vi "ColumbiaSonicareStby.vi"() -> ()   [LabVIEW 2022 SP3]
uses:
  Doppler data processing/Doppler/dopplerV6.llb/AI Waveform Scan (waveform).vi
  Doppler data processing/Doppler/dopplerV6.llb/AI Read (waveform).vi
  <vilib>/sound/lvsound.llb/Sound Format.ctl
panel:
  in  "Mode":enum32{"HIFU", "Thromb"}(tab)
  out "Exp Count":i32
  in  "Time between exposures (s)":sgl=2.2 min=0 format="%.1f"
  in  "Number of Exposures":i32=1 min=1
  in  "Therapy Duration (s)":dbl=0.1 min=0.1 max=10.0 step=0.1 format="%.1f"
  out "Time":i32=1 min=1
  out "PRF time  (ms)":sgl format="%.3f"
  in  "exp per cycle  (ms)":sgl=0.5 format="%.3f"
  in  "Total  Time On (s)":sgl=1.0 min=0.001 format="%.2f"
  out "PRF  (kHz)":sgl=1.0 min=0.001 format="%.3f"
  in  "Duty Cycle":sgl=0.5 min=0 max=1 format="%.2f"
  in  "EKG ?":bool=TRUE
  in  "Re-Zero Trig":bool
  out "waveform data":waveform(dbl)[](array[waveform])
  in  "New EKG (F1)":bool
  in  "Exit Program (F2)":bool
  out "EKG":waveform(dbl)[](graph)
  in  "Fire Therapy (ESC)":bool
  out "Therapy Delay (s)":dbl=1.0 format="%.3f"
  # "1. Select EKG mode with switch below.\n2. If in EKG mode, update EKG trace with New EKG (F1).\n3. Drag pink line to mark start time of exposure and trigger level.\n4. Set time duration of exposure (0.1 s steps).\n5. Choose number of exposures and time between exposures (2.2 s min in EKG mode)..\n6. Start exposure with Fire Therapy (ESC) (Green means on).\n7. Press Fire Therapy (ESC) again for emergency stop (Red means off).\n8. To exit program, Press Exit Program (F2) to  terminate program.\n9. Thromb tab permits exposures of a fixed PRF, duty cycle, and time duration. EKG  is\n     inactive when Thromb is selected."
  # "© 2003 Riverside Research Institute"
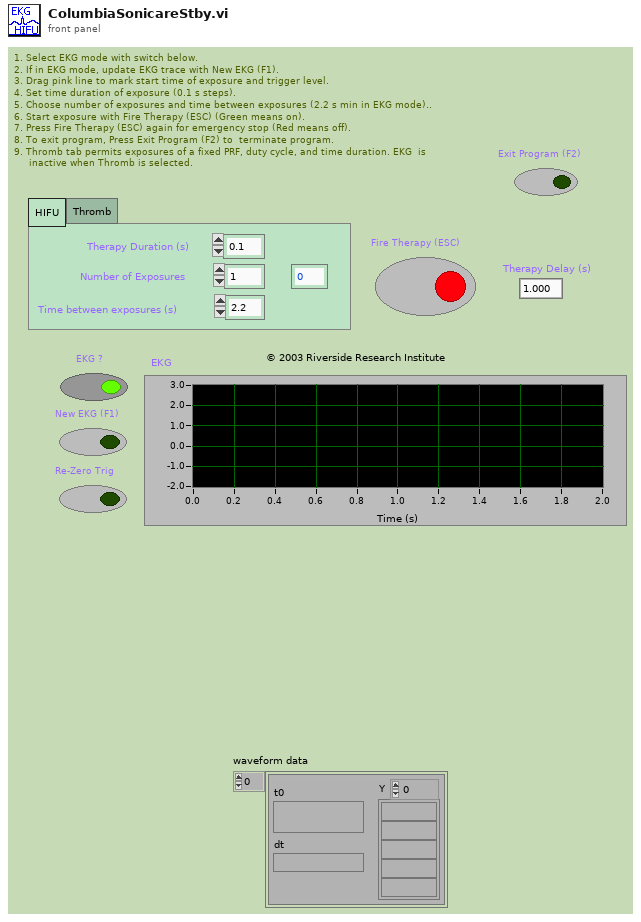
[diagram p1: front panel]
types:
  T1 = cluster{"coupling (no change:0)":enum16{"no change", "DC", "AC", "GND", "internal ref."}, "input config (no change:0)":u16}[]
  T2 = cluster{"high limit (0.0)":sgl, "low limit (0.0)":sgl}[]
  T3 = cluster{"trigger type (no trig:0)":enum16{"no trigger", "analog", "digital A", "digital B", "scan clock gate", "software analog "}, "pretrigger scans (0)":i32, "edge or slope \n(no change)":enum16{"no change", "rising", "falling"}, "analog chan (-) & level (0.0)":cluster{"trigger channel (empty)":string, "level (0.0)":sgl}, "scan clock source\n(no change:0)":enum16{"no change", "internal", "I/O Connector", "RTSI"}}
  T4 = typedef "Sound Format.ctl" = cluster{"sound quality":enum16{"mono", "stereo"}, "rate":enum16{"11025", "22050", "44100", "8000"}, "bits per sample":enum16{"8 bit", "16 bit"}}
  T5 = enum16{"ungated/software start", "count while high", "count while low", "start on rising edge", "start on falling edge"}
  T6 = enum16{"no trigger", "analog", "digital A", "digital A & B", "scan clock gate"}
  T7 = cluster{"trigger channel (empty)":string, "Cursor.Cursor Y":dbl}
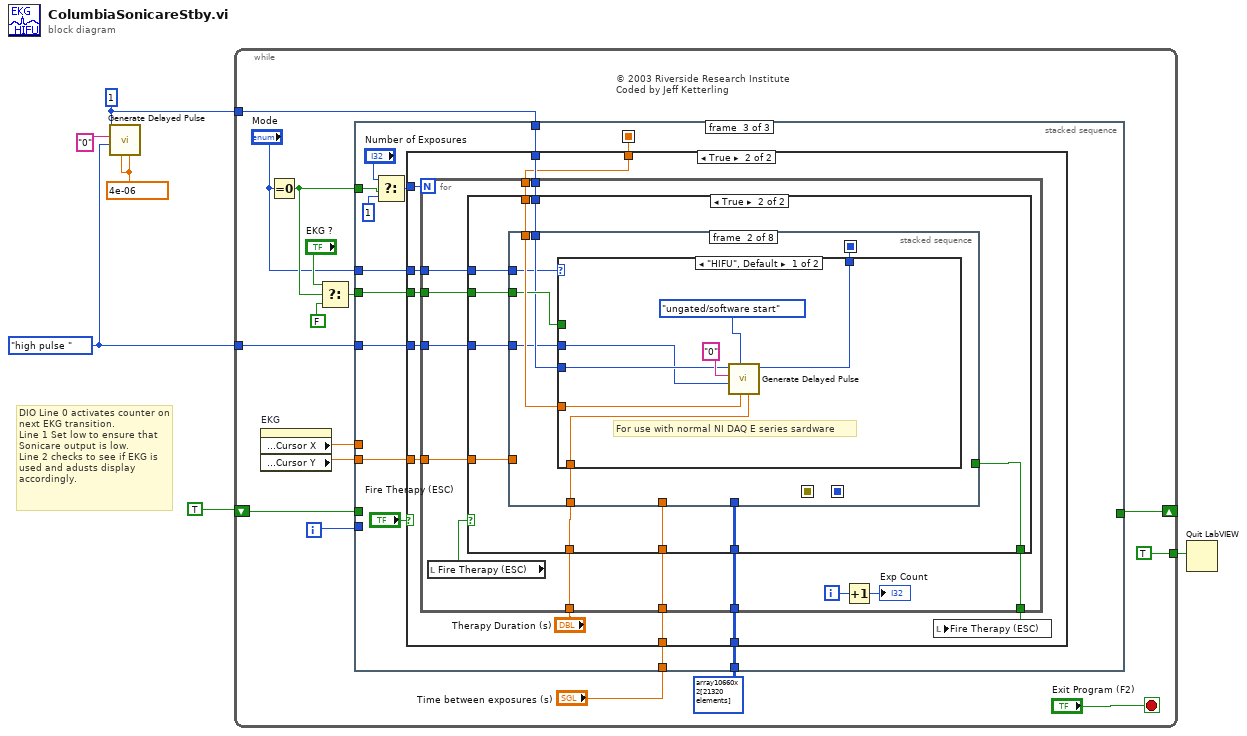
[diagram p0: block diagram]
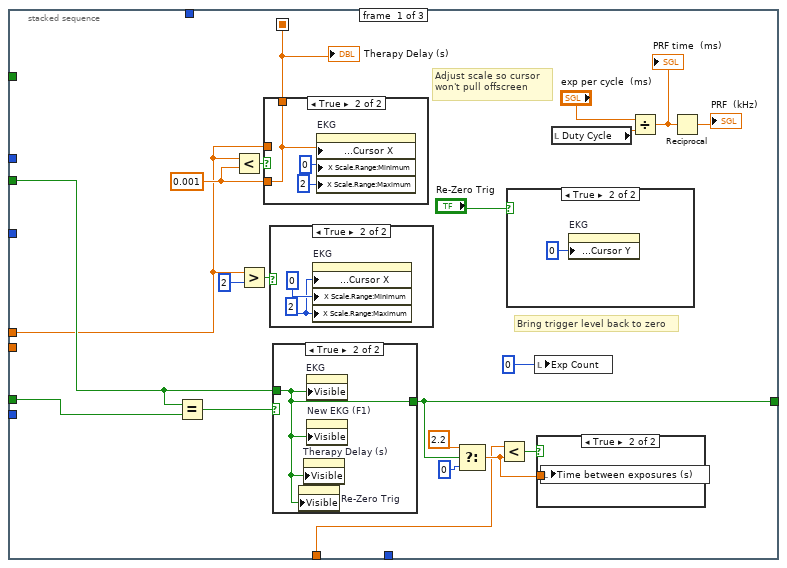
[diagram p2: hidden frame]
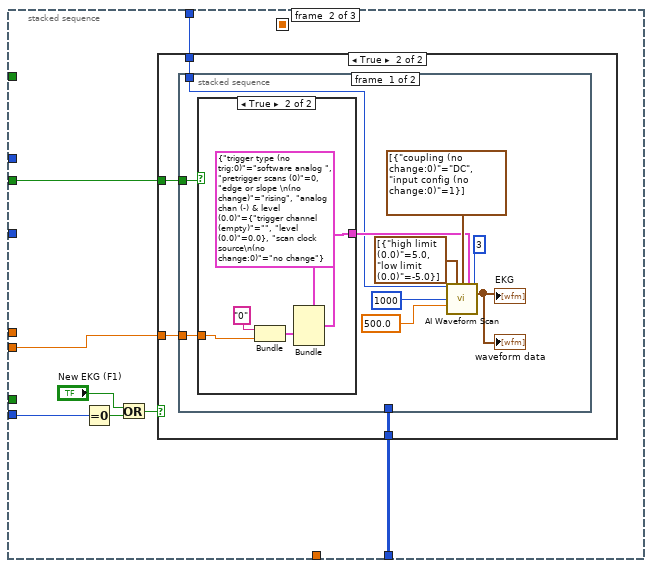
[diagram p8: hidden frame]
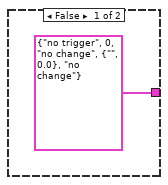
[diagram p10: hidden frame]
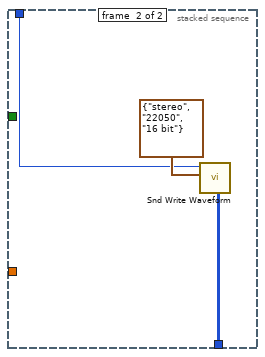
[diagram p11: hidden frame]
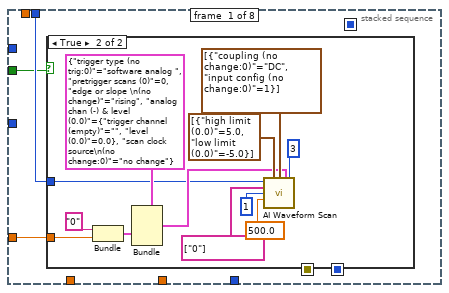
[diagram p14: hidden frame]
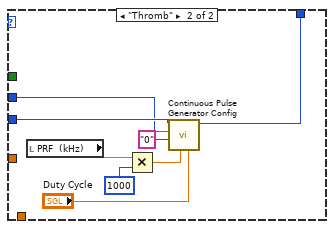
[diagram p16: hidden frame]
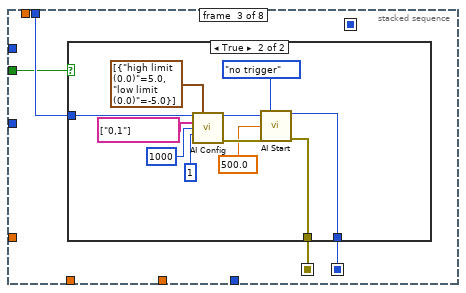
[diagram p17: hidden frame]
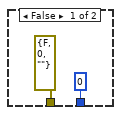
[diagram p18: hidden frame]
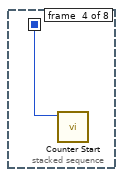
[diagram p19: hidden frame]
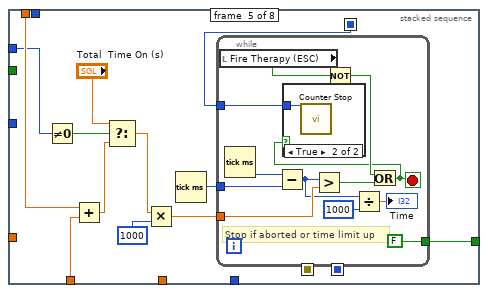
[diagram p20: hidden frame]
diagram:
  w2 = enum16{"high pulse ", "low pulse"}."high pulse " ("pulse polarity (high:0)")
  w3 = 4e-06
  w1 = 1
  # "DIO Line 0 activates counter on next EKG transition.\nLine 1 Set low to ensure that Sonicare output is low.\nLine 2 checks to see if EKG is used and adusts display accordingly."
  n1 = call <vilib>:"Generate Delayed Pulse.vi"("pulse width (s or cycles)"=w3, "pulse delay (s or cycles)"=w3, "pulse polarity (high:0)"=w2, "counter"="0", "device"=w1) -> ()  [unwired: 4 in, 3 out]
  n2 = while {
    tunnel: w1 -> [w18]
    shift-right: [w19] -> _
    shift-left: TRUE -> [w20]
    tunnel: [TRUE] -> w5
    tunnel: w2 -> [w7]
    i -> [w21]
    stop <- "Exit Program (F2)" stop-if-true
    # "© 2003 Riverside Research Institute\nCoded by Jeff Ketterling"
    n3 = property on="EKG" class="WFGraph (strict)"() -> ("Cursor.Cursor Position:Cursor X"=w15:dbl, "Cursor.Cursor Position:Cursor Y"=w16:dbl)  [unwired: 2 in, 2 out]
    n4 = Equal To 0?(x="Mode") -> (x = 0?=w9:bool)
    n5 = Select(t="EKG ?", s=w9, f=FALSE) -> (s? t:f=w11:bool)
    n6 = stacked-sequence {
      seq-local: [w42 _ _] -> [_ _ w95]
      tunnel: w18 -> [_ w61 w97]
      tunnel: w21 -> [_ w60 _]
      tunnel: w11 -> [w38 w56 w96]
      tunnel: w20 -> [w37 _ _]
      tunnel: [w29 _ _] -> w19
      tunnel: w16 -> [_ w55 w94]
      tunnel: w15 -> [w35 _ _]
      tunnel: i16[][] array10660x2[21320 elements] ("stereo 16-bit") -> [_ w54 w93]
      tunnel: "Time between exposures (s)" -> [w28 _ w92]
      tunnel: w9 -> [_ _ w89]
      tunnel: "Mode" -> [_ _ w86]
      tunnel: w7 -> [_ _ w85]
      frame #0 {
        w41 = 0.001
        # "Bring trigger level back to zero"
        # "Adjust scale so cursor won't pull offscreen"
        n7 = Equal?(x=w38, y=w37) -> (x = y?=w36:bool)
        n8 = Less?(x=w35, y=w41) -> (x < y?=w43:bool)
        n9 = Greater?(x=w35, y=2) -> (0:w39:bool)
        n10 = case shown="True" w43 {
          tunnel: w35 -> [w50 _]
          tunnel: [w50 w53] -> w42
          tunnel: w41 -> [_ w53]
          frame False {
          }
          frame True {
            n11 = property on="EKG" class="WFGraph (strict)"("Cursor.Cursor Position:Cursor X"=w53, "X Scale.Range:Minimum"=0, "X Scale.Range:Maximum"=2) -> ()  [unwired: 2 in, 2 out]
          }
        }
        "Therapy Delay (s)" <- w42
        n12 = case shown="True" w39 {
          frame False {
          }
          frame True {
            w48 = 2
            n13 = property on="EKG" class="WFGraph (strict)"("Cursor.Cursor Position:Cursor X"=w48, "X Scale.Range:Minimum"=0, "X Scale.Range:Maximum"=w48) -> ()  [unwired: 2 in, 2 out]
          }
        }
        n14 = case shown="True" w36 {
          tunnel: w38 -> [w46 w47]
          tunnel: [w46 w47] -> w29
          frame False {
          }
          frame True {
            n15 = property on="Re-Zero Trig" class="Bool"("Visible"=w47) -> ()  [unwired: 2 in, 2 out]
            n16 = property on="Therapy Delay (s)" class="DigNum (strict)"("Visible"=w47) -> ()  [unwired: 2 in, 2 out]
            n17 = property on="EKG" class="WFGraph (strict)"("Visible"=w47) -> ()  [unwired: 2 in, 2 out]
            n18 = property on="New EKG (F1)" class="Bool"("Visible"=w47) -> ()  [unwired: 2 in, 2 out]
          }
        }
        n19 = Select(t=2.2, s=w29, f=0) -> (s? t:f=w30:dbl)
        n20 = Less?(x=w28, y=w30) -> (x < y?=w31:bool)
        n21 = case shown="True" "Re-Zero Trig" {
          frame False {
          }
          frame True {
            n22 = property on="EKG" class="WFGraph (strict)"("Cursor.Cursor Position:Cursor Y"=0) -> ()  [unwired: 2 in, 2 out]
          }
        }
        n23 = local write "Exp Count"(0) -> ()
        n24 = case shown="True" w31 {
          tunnel: w30 -> [_ w44]
          frame False {
          }
          frame True {
            n25 = local write "Time between exposures (s)"(w44) -> ()
          }
        }
        n26 = local read "Duty Cycle"() -> (w26:sgl)
        n27 = Divide(x="exp per cycle  (ms)", y=w26) -> (x/y=w24:sgl)
        "PRF time  (ms)" <- w24
        n28 = Reciprocal(x=w24) -> (1/x=→"PRF  (kHz)":sgl)
      }
      frame #1 {
        n29 = Equal To 0?(x=w60) -> (x = 0?=w59:bool)
        n30 = Or(x="New EKG (F1)", y=w59) -> (x .or. y?=w57:bool)
        n31 = case shown="True" w57 {
          tunnel: w61 -> [_ w64]
          tunnel: w56 -> [_ w65]
          tunnel: w55 -> [_ w63]
          tunnel: w54 -> [_ w62]
          frame False {
          }
          frame True {
            n32 = stacked-sequence {
              tunnel: w65 -> [w68 _]
              tunnel: w64 -> [w67 w82]
              tunnel: w63 -> [w66 _]
              tunnel: w62 -> [_ w83]
              frame #0 {
                n33 = case shown="True" w68 {
                  tunnel: [T3 {"trigger type (no trig:0)"=enum."no trigger", "pretrigger scans (0)"=0, "edge or slope \n(no change)"=enum."no change", "analog chan (-) & level (0.0)"={"trigger channel (empty)"="", "level (0.0)"=0.0}, "scan clock source\n(no change:0)"=enum."no change"} ("trigger and clock (no trig, int clk)") w81] -> w70
                  tunnel: w66 -> [_ w80]
                  frame False {
                  }
                  frame True {
                    n34 = Bundle("trigger channel (empty)"="0", "Cursor.Cursor Y"=w80) -> (w78:T7)  [unwired: 1 in]
                    n35 = Bundle(cluster=T3 {"trigger type (no trig:0)"=enum."software analog ", "pretrigger scans (0)"=0, "edge or slope \n(no change)"=enum."rising", "analog chan (-) & level (0.0)"={"trigger channel (empty)"="", "level (0.0)"=0.0}, "scan clock source\n(no change:0)"=enum."no change"} ("trigger and clock (no trig, int clk)"), "analog chan (-) & level (0.0)"=w78) -> (w81:T3)  [unwired: 4 in]
                  }
                }
                n36 = call-poly "AI Waveform Scan.vi"("device (1)"=w67, "input limits (no change)"=T2 [{"high limit (0.0)"=5.0, "low limit (0.0)"=-5.0}], "coupling & input config (no change:0)"=T1 [{"coupling (no change:0)"=enum."DC", "input config (no change:0)"=1}], "trigger and clock (no trig, int clk)"=w70, "time limit in sec \n(computed:-1)"=3, "number of scans\n(1000)"=1000, "scan rate (1000 scans/sec)"=sgl 500.0) -> ("waveform data"=→"EKG" →"waveform data":waveform(dbl)[])  [unwired: 7 in, 1 out]
              }
              frame #1 {
                n37 = call <vilib>:"Snd Write Waveform.vi"("stereo 16-bit"=w83, "sound format"=T4 {"sound quality"=enum."stereo", "rate"=enum."22050", "bits per sample"=enum."16 bit"}, "device (0)"=w82) -> ()  [unwired: 8 in, 1 out]
              }
            }
          }
        }
      }
      frame #2 {
        n38 = Select(t="Number of Exposures", s=w89, f=1) -> (s? t:f=w87:i32)
        n39 = case shown="True" "Fire Therapy (ESC)" {
          tunnel: w97 -> [_ w108]
          tunnel: w96 -> [_ w107]
          tunnel: w95 -> [_ w106]
          tunnel: w87 -> [_ w105]
          tunnel: w94 -> [_ w104]
          tunnel: w93 -> [_ w102]
          tunnel: w92 -> [_ w101]
          tunnel: w86 -> [_ w99]
          tunnel: w85 -> [_ w98]
          frame False {
          }
          frame True {
            n40 = for {
              N: w105 -> [_]
              tunnel: w108 -> [w121]
              tunnel: w106 -> [w120]
              tunnel: w107 -> [w119]
              tunnel: w104 -> [w118]
              tunnel: [w117] -> w103
              tunnel: w102 -> [w116]
              tunnel: w101 -> [w114]
              tunnel: "Therapy Duration (s)" -> [w113]
              tunnel: w99 -> [w110]
              tunnel: w98 -> [w109]
              i -> [w115]
              n41 = local read "Fire Therapy (ESC)"() -> (w111:bool)
              n42 = case shown="True" w111 {
                selector: w111 -> [w122 _]
                tunnel: w121 -> [_ w132]
                tunnel: w120 -> [_ w131]
                tunnel: w119 -> [_ w130]
                tunnel: w118 -> [_ w129]
                tunnel: [w122 w128] -> w117
                tunnel: w116 -> [_ w127]
                tunnel: w114 -> [_ w126]
                tunnel: w113 -> [_ w125]
                tunnel: w110 -> [_ w124]
                tunnel: w109 -> [_ w123]
                frame False {
                }
                frame True {
                  n43 = stacked-sequence {
                    seq-local: [_ w151 _ _ _ _ _ _] -> [_ _ _ w187 w193 _ _ _]
                    seq-local: [_ _ w172 _ _ _ _ _] -> [_ _ _ _ _ w215 _ _]
                    seq-local: [_ _ w171 _ _ _ _ _] -> [_ _ _ _ _ w214 _ _]
                    tunnel: w132 -> [w135 w150 w173 _ _ _ w222 _]
                    tunnel: [_ _ _ _ w196 _ _ _] -> w128
                    tunnel: w131 -> [_ w154 _ _ w195 _ _ _]
                    tunnel: w125 -> [_ w153 _ _ w194 _ _ _]
                    tunnel: w130 -> [w134 w152 w170 _ _ w213 _ w227]
                    tunnel: w129 -> [w133 _ _ _ _ _ _ _]
                    tunnel: w127 -> [_ _ _ _ _ _ w223 _]
                    tunnel: w126 -> [_ _ _ _ _ _ _ w225]
                    tunnel: w124 -> [_ w149 _ _ w190 _ _ _]
                    tunnel: w123 -> [_ w148 _ _ _ _ _ _]
                    frame #0 {
                      n44 = case shown="True" w134 {
                        tunnel: w135 -> [_ w137]
                        tunnel: w133 -> [_ w138]
                        frame False {
                        }
                        frame True {
                          n45 = Bundle("trigger channel (empty)"="0", "Cursor.Cursor Y"=w138) -> (w139:T7)  [unwired: 1 in]
                          n46 = Bundle(cluster=T3 {"trigger type (no trig:0)"=enum."software analog ", "pretrigger scans (0)"=0, "edge or slope \n(no change)"=enum."rising", "analog chan (-) & level (0.0)"={"trigger channel (empty)"="", "level (0.0)"=0.0}, "scan clock source\n(no change:0)"=enum."no change"} ("trigger and clock (no trig, int clk)"), "analog chan (-) & level (0.0)"=w139) -> (w141:T3)  [unwired: 4 in]
                          n47 = call-poly "AI Waveform Scan.vi"("device (1)"=w137, "input limits (no change)"=T2 [{"high limit (0.0)"=5.0, "low limit (0.0)"=-5.0}], "coupling & input config (no change:0)"=T1 [{"coupling (no change:0)"=enum."DC", "input config (no change:0)"=1}], "trigger and clock (no trig, int clk)"=w141, "time limit in sec \n(computed:-1)"=3, "channels (0)"=tag[] ["0"], "number of scans\n(1000)"=1, "scan rate (1000 scans/sec)"=sgl 500.0) -> ()  [unwired: 6 in, 2 out]
                        }
                      }
                    }
                    frame #1 {
                      n48 = case shown="\"HIFU\", Default" w149 {
                        tunnel: w154 -> [w160 _]
                        tunnel: w153 -> [w159 _]
                        tunnel: w152 -> [_ _]
                        tunnel: [w158 w167] -> w151
                        tunnel: w150 -> [w157 w168]
                        tunnel: w148 -> [w155 w162]
                        frame "HIFU", Default {
                          # "For use with normal NI DAQ E series sardware"
                          n49 = call <vilib>:"Generate Delayed Pulse.vi"("pulse width (s or cycles)"=w159, "pulse delay (s or cycles)"=w160, "gate mode (ungated:0)"=T5."ungated/software start", "pulse polarity (high:0)"=w155, "counter"="0", "device"=w157) -> ("[taskID]"=w158:u32)  [unwired: 3 in, 2 out]
                        }
                        frame "Thromb" {
                          n50 = local read "PRF  (kHz)"() -> (w163:sgl)
                          n51 = Multiply(x=w163, y=1000) -> (x*y=w165:sgl)
                          n52 = call <vilib>:"Continuous Pulse Generator Config.vi"("duty cycle (0.5)"="Duty Cycle", "frequency (Hz)"=w165, "pulse polarity (high:0)"=w162, "counter"="0", "device"=w168) -> ("taskID"=w167:u32)  [unwired: 3 in, 3 out]
                        }
                      }
                    }
                    frame #2 {
                      n53 = case shown="True" w170 {
                        tunnel: w173 -> [_ w179]
                        tunnel: [u32 0 ("taskID out") w178] -> w172
                        tunnel: [errorcluster {"status"=FALSE, "code"=0, "source"=""} ("error out") w177] -> w171
                        frame False {
                        }
                        frame True {
                          n54 = call "AI Config.vi"("device (1)"=w179, "input limits (no change)"=T2 [{"high limit (0.0)"=5.0, "low limit (0.0)"=-5.0}], "channels (0)"=tag[] ["0,1"], "buffer size (1000 scans)"=1000, "[group] (0)"=1) -> ("taskID"=w181:u32, "error out"=w186:errorcluster)  [unwired: 8 in, 1 out]
                          n55 = call "AI Start.vi"("taskID in"=w181, "trigger type (no trig:0)"=T6."no trigger", "scan rate (1000 scans/sec)"=sgl 500.0, "error in (no error)"=w186) -> ("taskID out"=w178:u32, "error out"=w177:errorcluster)  [unwired: 8 in, 2 out]
                        }
                      }
                    }
                    frame #3 {
                      n56 = call <vilib>:"Counter Start.vi"("taskID"=w187) -> ()  [unwired: 9 in, 2 out]
                    }
                    frame #4 {
                      n57 = Not Equal To 0?(x=w190) -> (x != 0?=w192:bool)
                      n58 = Add(x=w195, y=w194) -> (x+y=w189:dbl)
                      n59 = Select(t="Total  Time On (s)", s=w192, f=w189) -> (s? t:f=w188:dbl)
                      n60 = Multiply(x=w188, y=1000) -> (x*y=w197:dbl)
                      n61 = Tick Count (ms)() -> (millisecond timer value=w199:u32)
                      n62 = while {
                        tunnel: w193 -> [w211]
                        tunnel: w199 -> [w209]
                        tunnel: w197 -> [w208]
                        tunnel: [FALSE] -> w196
                        stop <- w203 stop-if-true
                        # "Stop if aborted or time limit up"
                        n63 = local read "Fire Therapy (ESC)"() -> (w205:bool)
                        n64 = Tick Count (ms)() -> (millisecond timer value=w210:u32)
                        n65 = Subtract(x=w210, y=w209) -> (x-y=w202:u32)
                        n66 = Greater?(x=w202, y=w208) -> (0:w207:bool)
                        n67 = Not(x=w205) -> (.not. x?=w204:bool)
                        n68 = Divide(x=w202, y=1000) -> (x/y=→"Time":dbl)
                        n69 = Or(x=w204, y=w207) -> (x .or. y?=w203:bool)
                        n70 = case shown="True" w203 {
                          tunnel: w211 -> [_ w212]
                          frame False {
                          }
                          frame True {
                            n71 = call <vilib>:"Counter Stop.vi"("taskID"=w212) -> ()  [unwired: 5 in, 2 out]
                          }
                        }
                      }
                    }
                    frame #5 {
                      n72 = case shown="True" w213 {
                        tunnel: w215 -> [_ w217]
                        tunnel: w214 -> [_ w216]
                        frame False {
                        }
                        frame True {
                          n73 = call-poly "AI Read.vi"("taskID in"=w217, "number of scans to read (-1:all)"=1000, "error in (no error)"=w216) -> ("taskID out"=w220:u32, "waveform data"=w218:waveform(dbl)[], "error out"=w219:errorcluster)  [unwired: 7 in, 3 out]
                          n74 = local write "EKG"(w218) -> ()
                          n75 = call "AI Clear.vi"("error in (no error)"=w219, "taskID in"=w220) -> ()  [unwired: 4 in, 2 out]
                        }
                      }
                    }
                    frame #6 {
                      n76 = call <vilib>:"Snd Write Waveform.vi"("stereo 16-bit"=w223, "sound format"=T4 {"sound quality"=enum."stereo", "rate"=enum."22050", "bits per sample"=enum."16 bit"}, "device (0)"=w222) -> ()  [unwired: 8 in, 1 out]
                    }
                    frame #7 {
                      n77 = Select(t=2.2, s=w227, f=0) -> (s? t:f=w228:dbl)
                      n78 = Subtract(x=w225, y=w228) -> (x-y=w231:dbl)
                      n79 = Multiply(x=w231, y=1000) -> (x*y=w230:dbl)
                      n80 = Wait (ms)(milliseconds to wait=w230) -> ()  [unwired: 1 out]
                    }
                  }
                }
              }
              n81 = Increment(x=w115) -> (x+1=→"Exp Count":i32)
            }
            n82 = local write "Fire Therapy (ESC)"(w103) -> ()
          }
        }
      }
    }
  }
  n83 = Quit LabVIEW(quit? (T)=w5) -> ()
